vi "Packetizer.vi"(10 "TokenByte":u8, 11 "Data In":u8[](array[numeric])) -> (3 "Tokens":cluster{"Array 2":u8[]}[](array[cluster]))   [LabVIEW 2009]
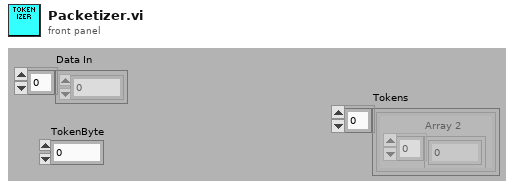
[diagram p1: front panel]
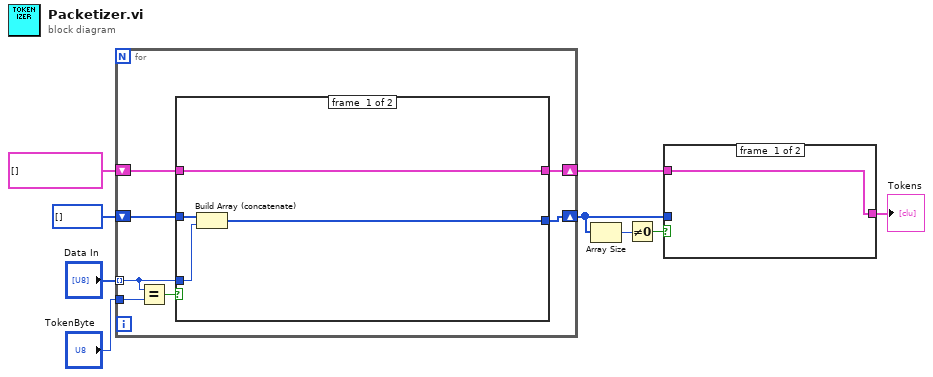
[diagram p0: block diagram]
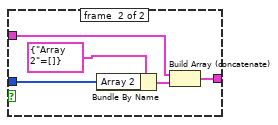
[diagram p2: hidden frame]
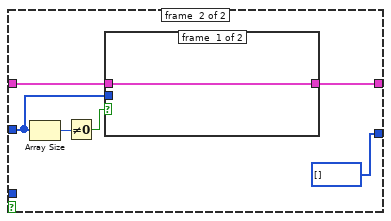
[diagram p3: hidden frame]
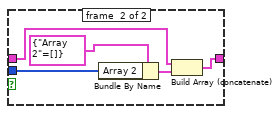
[diagram p4: hidden frame]
diagram:
  n1 = for {
    tunnel: "Data In" -> [w12] mode=indexing
    tunnel: "TokenByte" -> [w16]
    shift-right: [w14] -> w2
    shift-left: u8[] [] ("Array 2") -> [w13]
    shift-right: [w10] -> w3
    shift-left: cluster{"Array 2":u8[]}[] [] ("Tokens") -> [w11]
    n2 = Equal?(x=w12, y=w16) -> (x = y?=w15:bool)
    n3 = case shown="True" w15 {
      tunnel: [w18 u8[] [] ("Array 2")] -> w14
      tunnel: w13 -> [w20 w23]
      tunnel: w12 -> [w19 _]
      tunnel: w11 -> [w17 w22]
      tunnel: [w17 w21] -> w10
      frame #0 {
        n4 = Build Array (concatenate)(w20, w19) -> (w18:u8[])
      }
      frame #1 {
        n5 = Array Size(array=w23) -> (size(s)=w25:i32)
        n6 = Not Equal To 0?(x=w25) -> (x != 0?=w24:bool)
        n7 = case shown="False" w24 {
          tunnel: w23 -> [_ w31]
          tunnel: w22 -> [w27 w29]
          tunnel: [w27 w28] -> w21
          frame #0 {
          }
          frame #1 {
            n8 = Bundle By Name(cluster=cluster{"Array 2":u8[]} {"Array 2"=[]} ("Cluster"), "Array 2"=w31) -> (w30:cluster{"Array 2":u8[]})
            n9 = Build Array (concatenate)(w29, w30) -> (w28:cluster{"Array 2":u8[]}[])
          }
        }
      }
    }
  }
  n10 = Array Size(array=w2) -> (size(s)=w5:i32)
  n11 = Not Equal To 0?(x=w5) -> (x != 0?=w4:bool)
  n12 = case shown="False" w4 {
    tunnel: w2 -> [_ w37]
    tunnel: w3 -> [w33 w35]
    tunnel: [w33 w34] -> w1
    frame #0 {
    }
    frame #1 {
      n13 = Bundle By Name(cluster=cluster{"Array 2":u8[]} {"Array 2"=[]} ("Cluster"), "Array 2"=w37) -> (w36:cluster{"Array 2":u8[]})
      n14 = Build Array (concatenate)(w35, w36) -> (w34:cluster{"Array 2":u8[]}[])
    }
  }
  "Tokens" <- w1
